vi "SendMessage.vi"(8 "error in (no error)":errorcluster, 9 "Parameters":variant, 10 "Destination":variant, 11 "AppLogger.Message.Log in":refnum<class "AppLogger.Message.Log.lvclass">) -> (0 "error out":errorcluster, 3 "AppLogger.Message.Log out":refnum<class "AppLogger.Message.Log.lvclass">)   [LabVIEW 2014, in "AppLogger.Message.Log.lvclass"]
uses:
  AppLogger.Message.Log.lvclass
  AppLogger.lvclass
panel:
  in  "AppLogger.lvclass":refnum<class "AppLogger.lvclass">
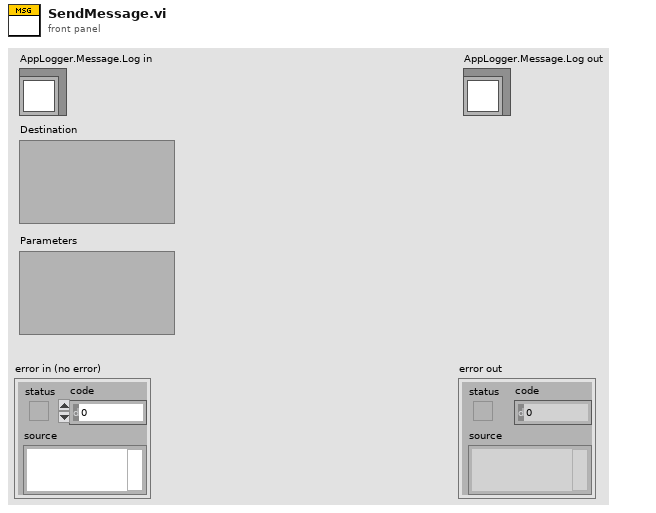
[diagram p1: front panel]
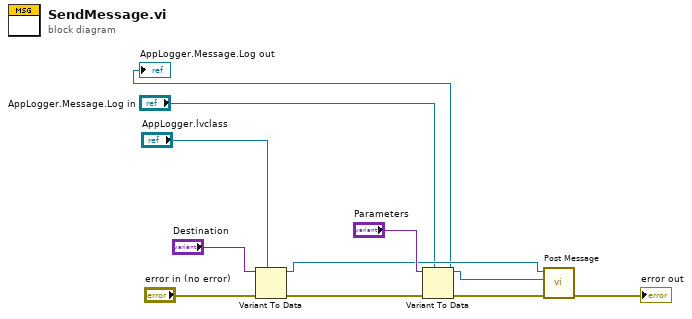
[diagram p0: block diagram]
diagram:
  n1 = Variant To Data(error in="error in (no error)", type="AppLogger.lvclass", Variant="Destination") -> (data=w5:refnum<class "AppLogger.lvclass">, error out=w6:errorcluster)
  n2 = Variant To Data(error in=w6, type="AppLogger.Message.Log in", Variant="Parameters") -> (data=w1:refnum<class "AppLogger.Message.Log.lvclass">, error out=w4:errorcluster)
  "AppLogger.Message.Log out" <- w1
  n3 = call-dynamic "Post Message.vi"("error in (no error)"=w4, "Message in"=w1, "Messenger in"=w5) -> ("error out"=→"error out":errorcluster)  [unwired: 7 in, 1 out]
